vi "linear interpolation - complex.vi"(7 "n":i32=-1, 11 "Array":cdb[](array[numeric])) -> (0 "interpolated average":cdb, 1 "mean":cdb, 2 "sum n z_n":cdb, 3 "sum z_n":cdb, 4 "slope":cdb, 5 "sigma":dbl, 6 "intercept":cdb)   [LabVIEW 2015]
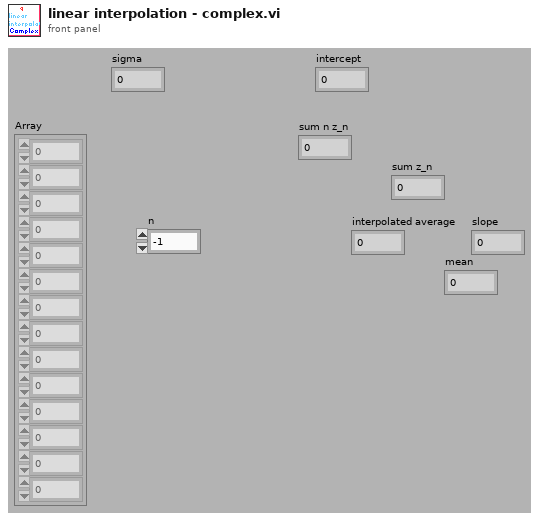
[diagram p1: front panel]
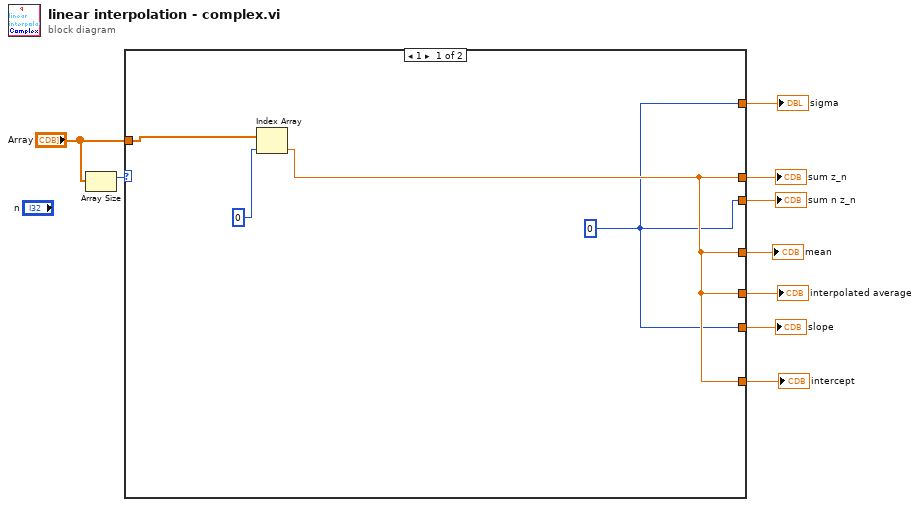
[diagram p0: block diagram]
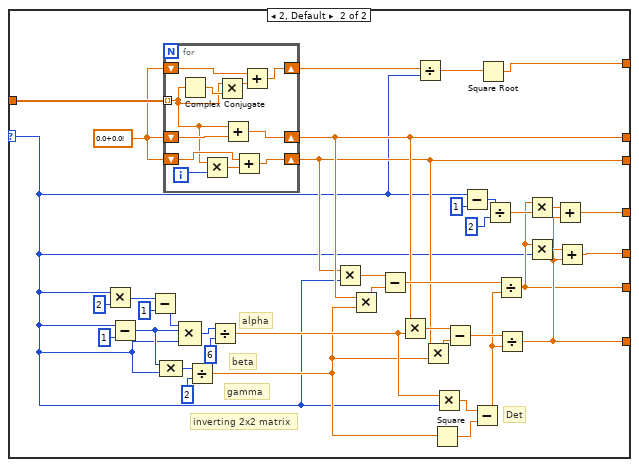
[diagram p2: hidden frame]
diagram:
  n1 = Array Size(array="Array") -> (size(s)=w2:i32)
  n2 = case shown="1" w2 {
    selector: w2 -> [_ w16]
    tunnel: [w11 w25] -> w9
    tunnel: [w10 w24] -> w8
    tunnel: [w11 w23] -> w7
    tunnel: [w11 w22] -> w6
    tunnel: [w11 w21] -> w5
    tunnel: [w10 w20] -> w4
    tunnel: "Array" -> [w13 w19]
    tunnel: [w10 w14] -> w1
    frame 1 {
      w10 = 0 ("index")
      n3 = Index Array(array=w13, index=0) -> (element=w11:cdb)
    }
    frame 2, Default {
      w18 = cdb 0.0+0.0i
      # "inverting 2x2 matrix"
      # "Det"
      # "beta"
      # "gamma"
      # "alpha"
      n4 = Multiply(x=w16, y=2 ("n")) -> (x*y=w49:i32)
      n5 = Subtract(x=w16, y=1 ("n")) -> (x-y=w45:i32)
      n6 = Subtract(x=w49, y=1 ("n")) -> (x-y=w48:i32)
      n7 = Compound Arithmetic op=MULTIPLY(w45, w16) -> (w43:i32)
      n8 = for {
        tunnel: w19 -> [w53] mode=indexing
        shift-right: [w63] -> w21
        shift-left: w18 -> [w62]
        shift-right: [w60] -> w20
        shift-left: w18 -> [w58]
        shift-right: [w57] -> w17
        shift-left: w18 -> [w55]
        i -> [w59]
        n9 = Complex Conjugate(1:w53) -> (0:w56:cdb)
        n10 = Multiply(x=w53, y=w59) -> (x*y=w61:cdb)
        n11 = Multiply(x=w53, y=w56) -> (x*y=w54:cdb)
        n12 = Add(x=w53, y=w62) -> (x+y=w63:cdb)
        n13 = Add(x=w58, y=w61) -> (x+y=w60:cdb)
        n14 = Add(x=w55, y=w54) -> (x+y=w57:cdb)
      }
      n15 = Compound Arithmetic op=MULTIPLY(w48, w45, w16) -> (w47:i32)
      n16 = Divide(x=w43, y=2 ("n")) -> (x/y=w34:dbl)
      n17 = Divide(x=w47, y=6 ("n")) -> (x/y=w35:dbl)
      n18 = Multiply(x=w20, y=w16) -> (x*y=w39:cdb)
      n19 = Multiply(x=w21, y=w34) -> (x*y=w40:cdb)
      n20 = Subtract(x=w39, y=w40) -> (x-y=w38:cdb)
      n21 = Multiply(x=w21, y=w35) -> (x*y=w36:cdb)
      n22 = Divide(x=w17, y=w16) -> (x/y=w15:cdb)
      n23 = Multiply(x=w20, y=w34) -> (x*y=w37:cdb)
      n24 = Square(x=w34) -> (x^2=w41:dbl)
      n25 = Multiply(x=w35, y=w16) -> (x*y=w42:dbl)
      n26 = Subtract(x=w36, y=w37) -> (x-y=w33:cdb)
      n27 = Subtract(x=w16, y=1 ("n")) -> (x-y=w30:i32)
      n28 = Subtract(x=w42, y=w41) -> (x-y=w32:dbl)
      n29 = Square Root(x=w15) -> (sqrt(x)=w14:cdb)
      n30 = Divide(x=w30, y=2 ("n")) -> (x/y=w28:dbl)
      n31 = Divide(x=w38, y=w32) -> (x/y=w24:cdb)
      n32 = Divide(x=w33, y=w32) -> (x/y=w25:cdb)
      n33 = Multiply(x=w24, y=w28) -> (x*y=w27:cdb)
      n34 = Multiply(x=w24, y=w16) -> (x*y=w26:cdb)
      n35 = Add(x=w27, y=w25) -> (x+y=w22:cdb)
      n36 = Add(x=w26, y=w25) -> (x+y=w23:cdb)
    }
  }
  "interpolated average" <- w7
  "slope" <- w8
  "mean" <- w6
  "intercept" <- w9
  "sum n z_n" <- w4
  "sum z_n" <- w5
  "sigma" <- w1
